vi "Report.vi"() -> ()   [LabVIEW 2017]
uses:
  <vilib>/Utility/miscctls.llb/LVRowAndColumnUnsignedTypeDef.ctl
  a160b8e7-0040-4e34-a052-5f80b3aab475.vi
  <vilib>/addons/database/Connection.llb/DB Tools Open Connec (String).vi
  <vilib>/Utility/file.llb/Write Delimited Spreadsheet (string).vi
  Global/Global 1.vi
  <vilib>/addons/database/NI_Database_API.lvlib
  <vilib>/Utility/NIReport.llb/NI_report.lvclass
  <vilib>/Utility/NIReport.llb/Append Text Table to Report (wrap).vi
panel:
  out "reposr save header":string[](array[string])
  in  "SELECT REPORT TYPE":string(combo)="WITH TRECIABILITY"
  out "error out":errorcluster
  in  "error in (no error)":errorcluster
  in  "GET REPORT":bool
  in  "EXIT":bool
  in  "EXPORT TO EXCEL":bool
  in  "TO":timestamp format="%<%x>T"
  in  "FROM":timestamp format="%<%x>T"
  in  "BARCODE":string
  in  "TYPE":string(combo)="DATE TIME"
  in  "STATION WISE":string(combo)="OP 10"
  out "Table":string[][](table)
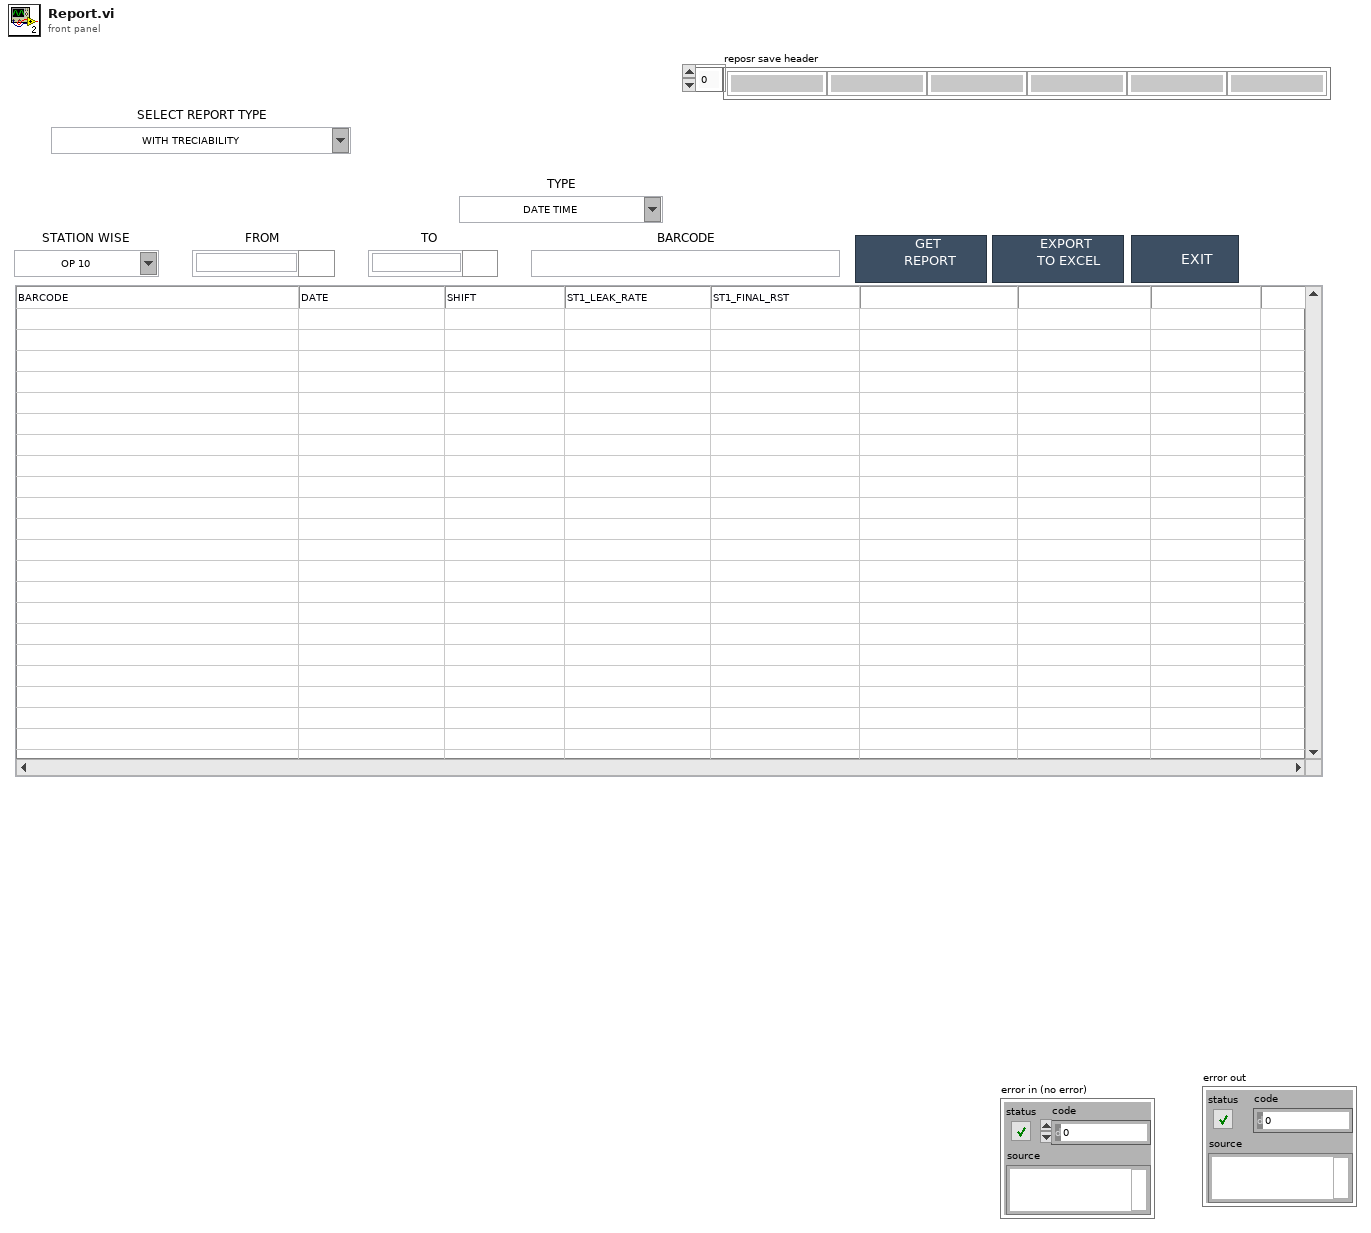
[diagram p1: front panel]
types:
  T1 = typedef "NI_Database_API.lvlib/Conn ObjectReference.ctl" = refnum<k1>
  T2 = typedef "LVRowAndColumnUnsignedTypeDef.ctl" = cluster{"Row":u32, "Column":u32}
  T3 = enum16{"Standard Report", "HTML", "Word", "Excel"}
  T4 = enum16{"maximized", "minimized", "normal", "no change"}
  T5 = typedef "LVRowAndColumnTypeDef.ctl" = cluster{"Row":i32, "Column":i32}
  T6 = enum32{"invalid app kind", "Development System", "Run Time System", "Student Edition", "Embedded LabVIEW", "Evaluation", "Custom"}
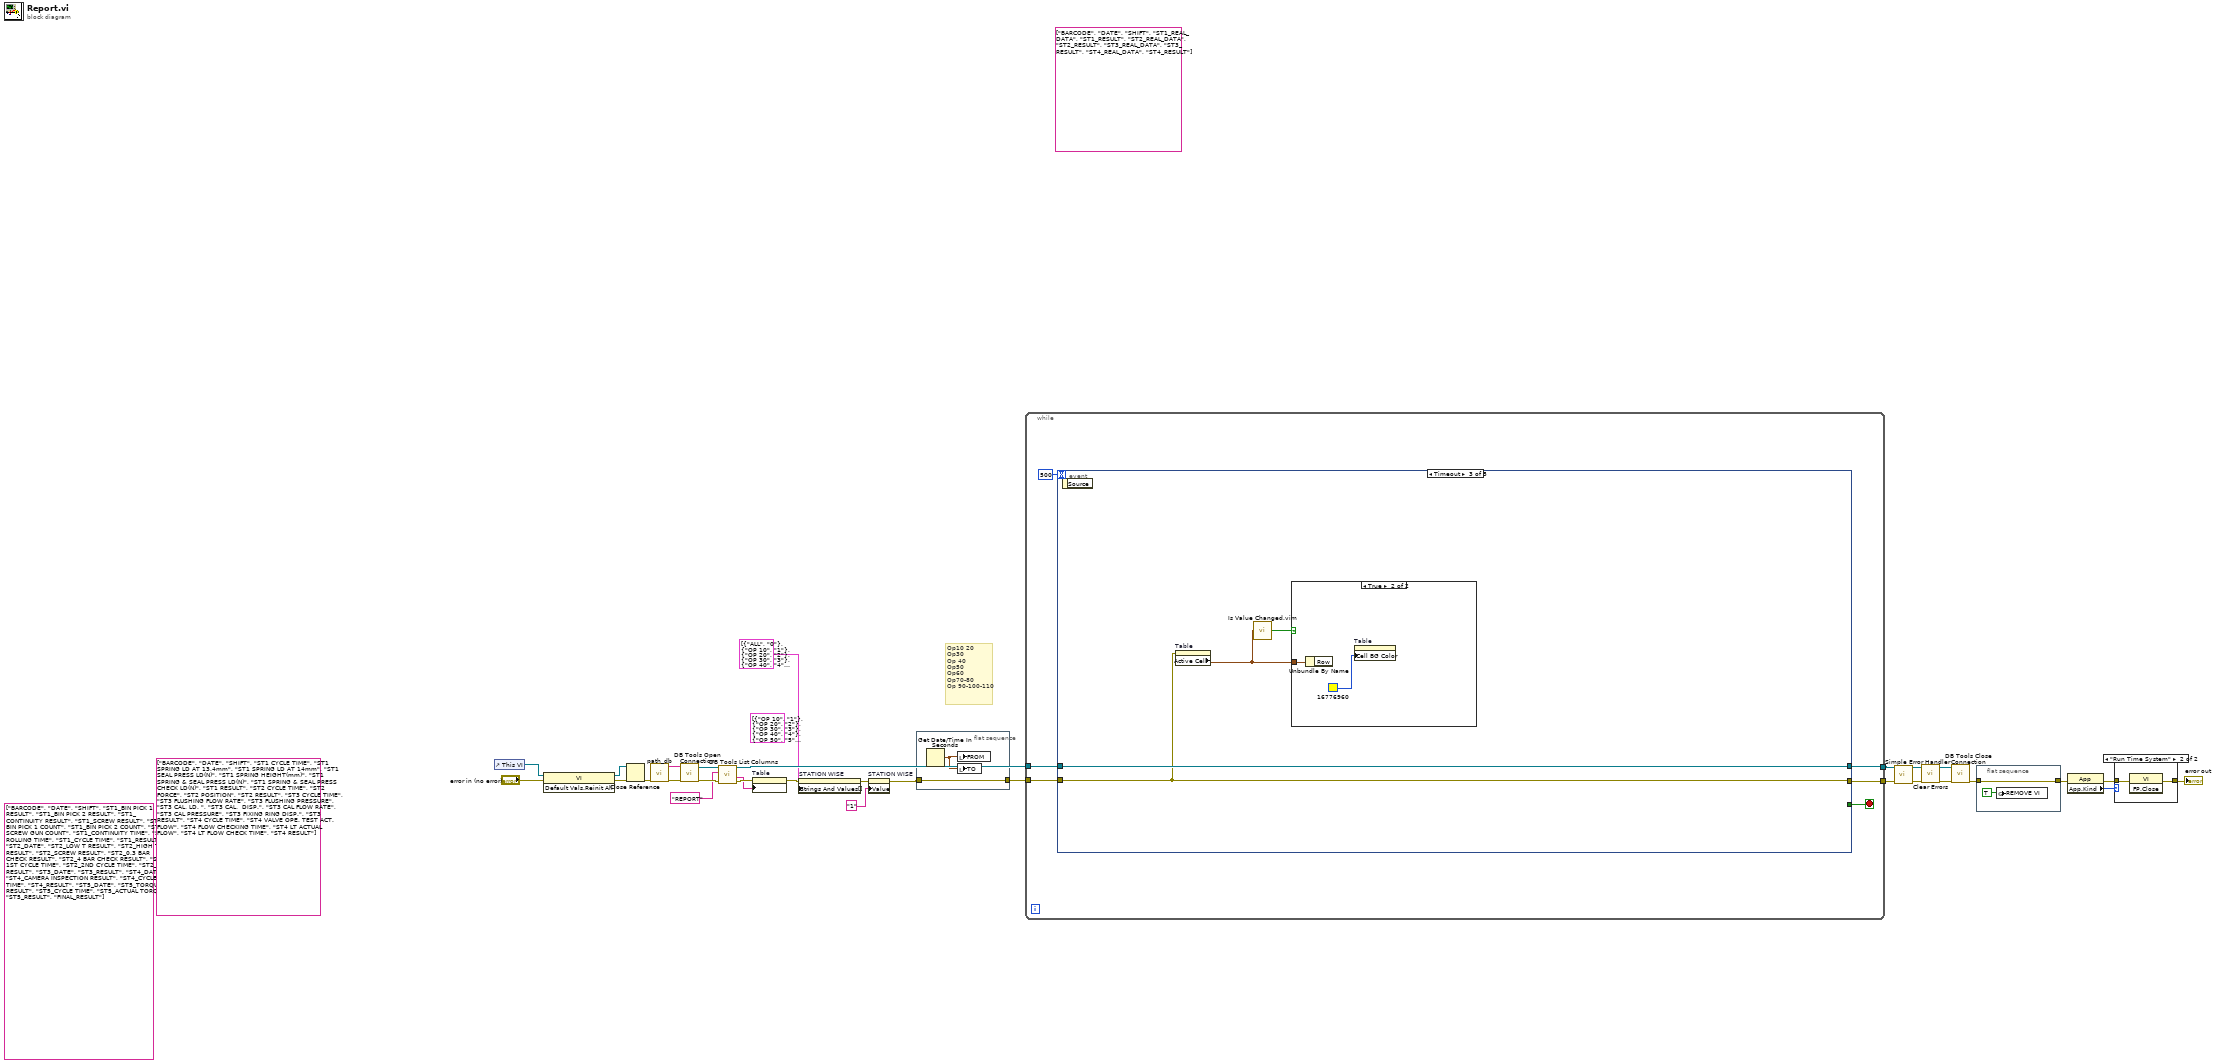
[diagram p0: block diagram]
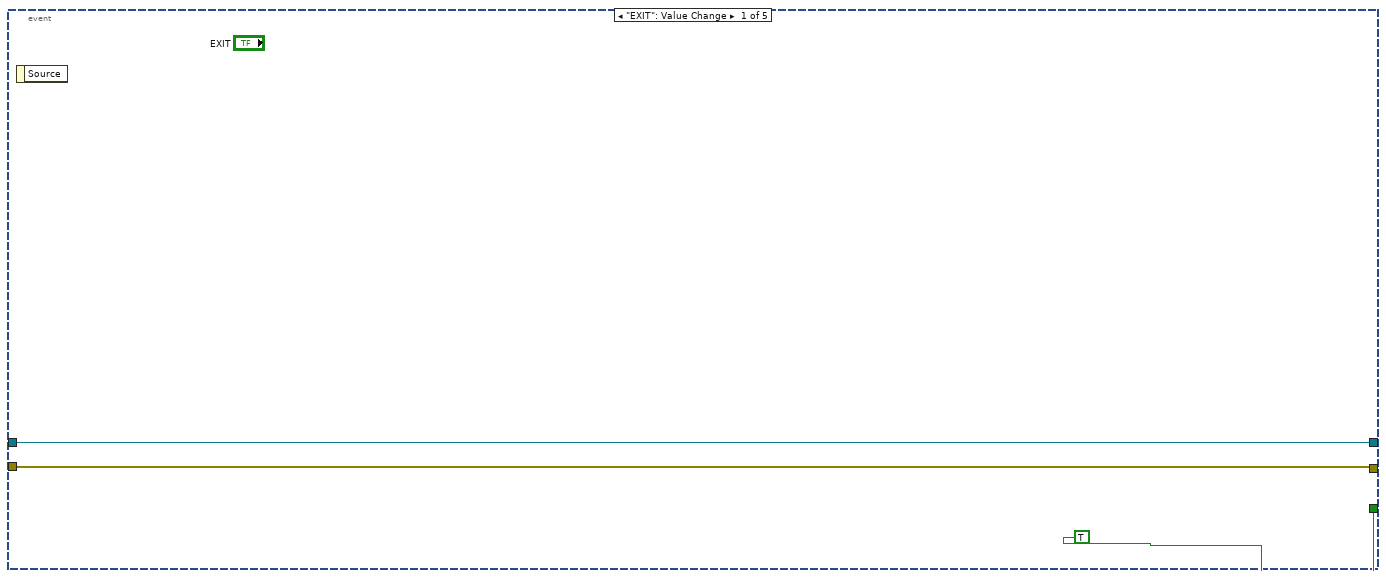
[diagram p2: hidden frame]
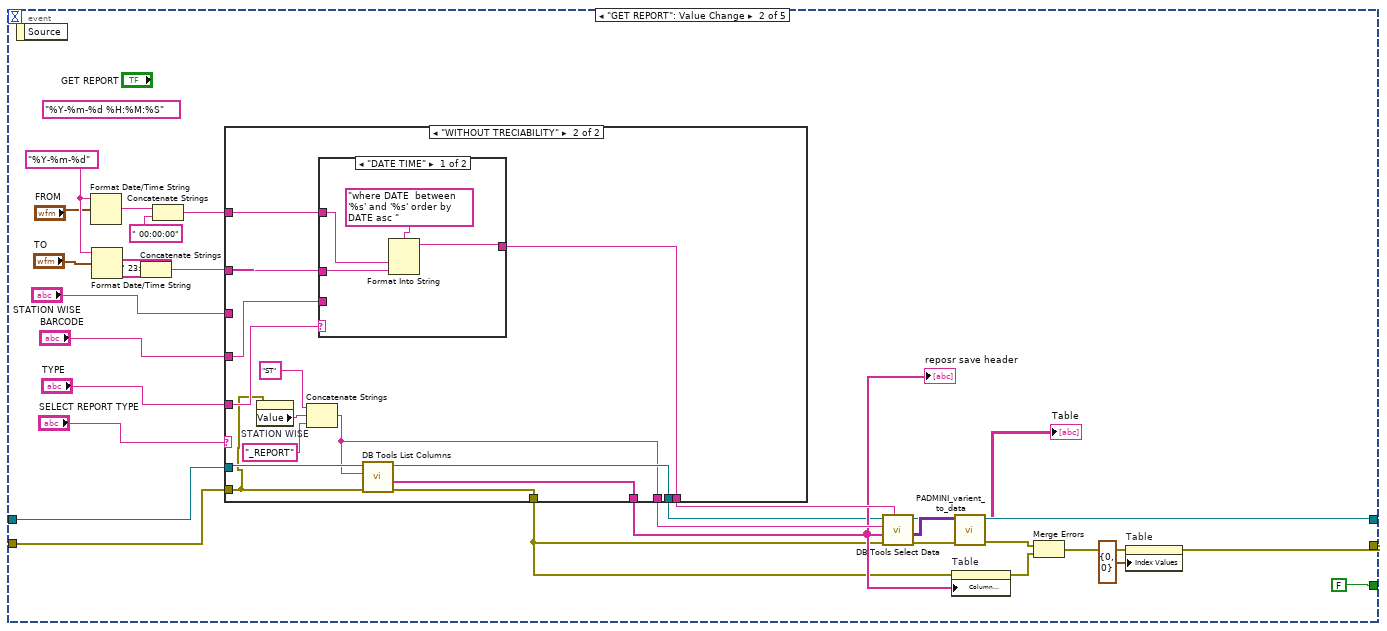
[diagram p3: hidden frame]
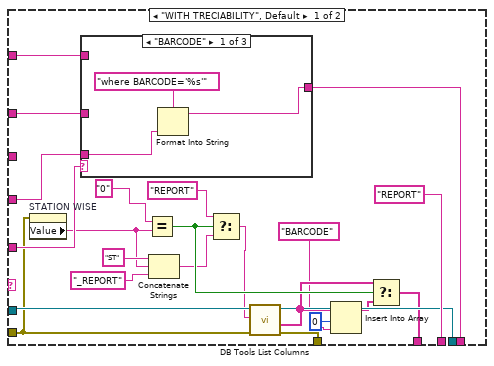
[diagram p4: hidden frame]
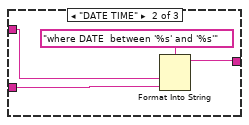
[diagram p5: hidden frame]
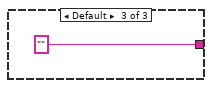
[diagram p6: hidden frame]
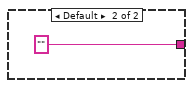
[diagram p7: hidden frame]
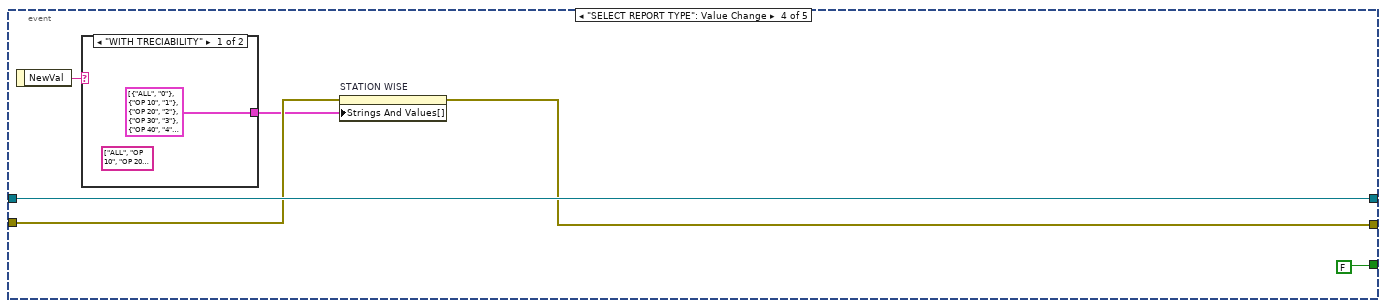
[diagram p9: hidden frame]
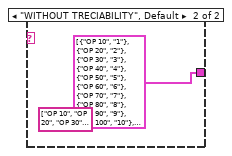
[diagram p10: hidden frame]
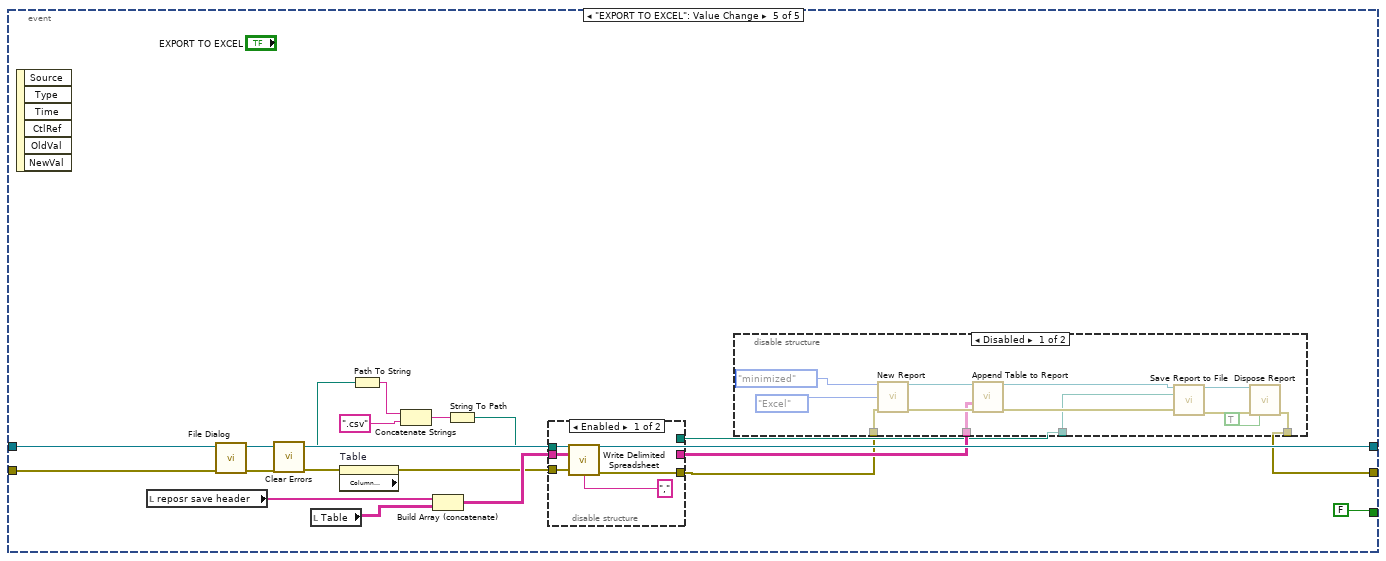
[diagram p11: hidden frame]
diagram:
  (unwired) cluster{"String":string, "Value":string}[] [{"String"="OP 10", "Value"="1"}, {"String"="OP 20", "Value"="2"}, {"String"="OP 30", "Value"="3"}, {"String"="OP 40", "Value"="4"}, {"String"="OP 50", "Value"="5"}, {"String"="OP 60", "Value"="6"}, {"String"="OP 70", "Value"="7"}, {"String"="OP 80", "Value"="8"}, {"String"="OP 90", "Value"="9"}, {"String"="OP 100", "Value"="10"}, {"String"="OP 110", "Value"="11"}] ("Strings And Values [] 2")
  (unwired) string[] ["BARCODE", "DATE", "SHIFT", "ST1_REAL_DATA", "ST1_RESULT", "ST2_REAL_DATA", "ST2_RESULT", "ST3_REAL_DATA", "ST3_RESULT", "ST4_REAL_DATA", "ST4_RESULT"]
  (unwired) string[] ["BARCODE", "DATE", "SHIFT", "ST1_BIN PICK 1 RESULT", "ST1_BIN PICK 2 RESULT", "ST1_CONTINUITY RESULT", "ST1_SCREW RESULT", "ST1_BIN PICK 1 COUNT", "ST1_BIN PICK 2 COUNT", "ST1_SCREW GUN COUNT", "ST1_CONTINUITY TIME", "ST1_ROLLING TIME", "ST1_CYCLE TIME", "ST1_RESULT", "ST2_DATE", "ST2_LOW T RESULT", "ST2_HIGH T RESULT", "ST2_SCREW RESULT", "ST2_0.3 BAR CHECK RESULT", "ST2_4 BAR CHECK RESULT", "ST2_1ST CYCLE TIME", "ST2_2ND CYCLE TIME", "ST2_RESULT", "ST3_DATE", "ST3_RESULT", "ST4_DATE", "ST4_CAMERA INSPECTION RESULT", "ST4_CYCLE TIME", "ST4_RESULT", "ST5_DATE", "ST5_TORQUE RESULT", "ST5_CYCLE TIME", "ST5_ACTUAL TORQUE", "ST5_RESULT", "FINAL_RESULT"]
  (unwired) string[] ["BARCODE", "DATE", "SHIFT", "ST1 CYCLE TIME", "ST1 SPRING LD AT 13.4mm", "ST1 SPRING LD AT 14mm", "ST1 SEAL PRESS LD(N)", "ST1 SPRING HEIGHT(mm)", "ST1 SPRING & SEAL PRESS LD(N)", "ST1 SPRING & SEAL PRESS CHECK LD(N)", "ST1 RESULT", "ST2 CYCLE TIME", "ST2 FORCE", "ST2 POSITION", "ST2 RESULT", "ST3 CYCLE TIME", "ST3 FLUSHING FLOW RATE", "ST3 FLUSHING PRESSURE", "ST3 CAL. LD. ", "ST3 CAL.  DISP.", "ST3 CAL FLOW RATE", "ST3 CAL PRESSURE", "ST3 FIXING RING DISP.", "ST3 RESULT", "ST4 CYCLE TIME", "ST4 VALVE OPE. TEST ACT. FLOW", "ST4 FLOW CHECKING TIME", "ST4 LT ACTUAL FLOW", "ST4 LT FLOW CHECK TIME", "ST4 RESULT"]
  # "Op10 20\nOp30\nOp 40\nOp50\nOp60\nOp70-80\nOp 90-100-110"
  n1 = control-ref of="This VI"() -> (w28:refnum<vi>)
  n2 = invoke class="VI" method="Default Vals.Reinit All"(reference=w28, error in="error in (no error)") -> (reference out=w26:refnum<vi>, error out=w25:errorcluster)  [unwired: 1 in, 1 out]
  n3 = Close Reference(reference=w26, error in (no error)=w25) -> (error out=w15:errorcluster)
  n4 = call "path_db.vi"("error in"=w15) -> ("error out"=w17:errorcluster, "resulting string"=w16:string)  [unwired: 9 in]
  n5 = call-poly <vilib>:"DB Tools Open Connection.vi"("error in (no error)"=w17, "connection information"=w16) -> ("error out"=w10:errorcluster, "connection reference"=w7:T1)  [unwired: 6 in]
  n6 = call <vilib>:"DB Tools List Columns.vi"("error in (no error)"=w10, "table"="REPORT", "connection reference"=w7) -> ("error out"=w9:errorcluster, "columns"=w6:string[], "connection reference out"=w8:T1)  [unwired: 1 in, 1 out]
  n7 = property on="Table" class="Tbl (strict)"(error in=w9, "Column Headers[]"=w6) -> (error out=w12:errorcluster)  [unwired: 1 in, 1 out]
  n8 = property on="STATION WISE" class="CmbBox"(error in=w12, "Strings And Values[]"=cluster{"String":string, "Value":string}[] [{"String"="ALL", "Value"="0"}, {"String"="OP 10", "Value"="1"}, {"String"="OP 20", "Value"="2"}, {"String"="OP 30", "Value"="3"}, {"String"="OP 40", "Value"="4"}, {"String"="OP 50", "Value"="5"}, {"String"="OP 60", "Value"="6"}, {"String"="OP 70", "Value"="7"}, {"String"="OP 80", "Value"="8"}, {"String"="OP 90", "Value"="9"}, {"String"="OP 100", "Value"="10"}, {"String"="OP 110", "Value"="11"}] ("Strings And Values [] 2")) -> (error out=w4:errorcluster)  [unwired: 1 in, 1 out]
  n9 = property on="STATION WISE" class="CmbBox"(error in=w4, "Value"="1") -> (error out=w3:errorcluster)  [unwired: 1 in, 1 out]
  n10 = flat-sequence {
    tunnel: w3 -> [w29]
    tunnel: [w29] -> w11
    frame #0 {
      n11 = Get Date/Time In Seconds() -> (seconds since 1Jan1904=w30:timestamp)
      n12 = local write "FROM"(w30) -> ()
      n13 = local write "TO"(w30) -> ()
    }
  }
  n14 = while {
    tunnel: [w33] -> w18
    tunnel: w11 -> [w35]
    tunnel: w8 -> [w34]
    tunnel: [w32] -> w13
    stop <- w36 stop-if-true
    n15 = event shown="[2] Timeout" {
      selector: _ -> [_ _ _ _ _]
      dyn-events: _ -> [_ _ _ _ _]
      timeout: 500 -> [_ _ _ _ _]
      tunnel: [TRUE FALSE _ FALSE FALSE] -> w36
      tunnel: w35 -> [w37 w46 w120 w129 w139]
      tunnel: w34 -> [w38 w44 w123 w131 w150]
      tunnel: [w38 w52 w123 w131 w150] -> w32
      tunnel: [w37 w53 w120 w126 w136] -> w33
      event "EXIT": Value Change {
        n16 = event-data() -> ()  [unwired: 1 in, 1 out]
      }
      event "GET REPORT": Value Change {
        (unwired) "%Y-%m-%d %H:%M:%S" ("time format string (%c)")
        w66 = "%Y-%m-%d" ("time format string (%c)")
        n17 = event-data() -> ()  [unwired: 1 in, 1 out]
        n18 = Format Date/Time String(time format string (%c)=w66, seconds (now)="FROM") -> (date/time string=w60:string)  [unwired: 1 in]
        n19 = Format Date/Time String(time format string (%c)=w66, seconds (now)="TO") -> (date/time string=w57:string)  [unwired: 1 in]
        n20 = Concatenate Strings(w57, " 23:59:59" ("time format string (%c)")) -> (w56:string)
        n21 = Concatenate Strings(w60, " 00:00:00" ("time format string (%c)")) -> (w59:string)
        n22 = case shown="\"WITHOUT TRECIABILITY\"" "SELECT REPORT TYPE" {
          tunnel: "TYPE" -> [w92 w114]
          tunnel: [w91 w113] -> w68
          tunnel: "BARCODE" -> [w90 w112]
          tunnel: w59 -> [w89 w111]
          tunnel: w56 -> [w88 w107]
          tunnel: "STATION WISE" -> [_ _]
          tunnel: ["REPORT" w102] -> w47
          tunnel: w46 -> [w70 w101]
          tunnel: [w84 w106] -> w40
          tunnel: [w80 w105] -> w45
          tunnel: w44 -> [w86 w104]
          tunnel: [w85 w103] -> w43
          frame "WITH TRECIABILITY", Default {
            n23 = property on="STATION WISE" class="CmbBox"(error in=w70) -> ("Value"=w71:string)  [unwired: 1 in, 2 out]
            n24 = case shown="\"BARCODE\"" w92 {
              tunnel: [w94 w98 ""] -> w91
              tunnel: w90 -> [w93 _ _]
              tunnel: w89 -> [_ w97 _]
              tunnel: w88 -> [_ w96 _]
              frame "BARCODE" {
                n25 = Format Into String(format string="where BARCODE='%s'", w93) -> (resulting string=w94:string)  [unwired: 2 in, 1 out]
              }
              frame "DATE TIME" {
                n26 = Format Into String(format string="where DATE  between '%s' and '%s'", w97, w96) -> (resulting string=w98:string)  [unwired: 2 in, 1 out]
              }
              frame Default {
              }
            }
            n27 = Equal?(x="0", y=w71) -> (x = y?=w82:bool)
            n28 = Concatenate Strings("ST", w71, "_REPORT") -> (w74:string)
            n29 = Select(t="REPORT", s=w82, f=w74) -> (s? t:f=w81:string)
            n30 = call <vilib>:"DB Tools List Columns.vi"("error in (no error)"=w70, "table"=w81, "connection reference"=w86) -> ("error out"=w84:errorcluster, "columns"=w79:string[], "connection reference out"=w85:T1)  [unwired: 1 in, 1 out]
            n31 = Insert Into Array(array=w79, index=0, new element="BARCODE" ("String")) -> (w77:string[])
            n32 = Select(t=w79, s=w82, f=w77) -> (s? t:f=w80:string[])
          }
          frame "WITHOUT TRECIABILITY" {
            n33 = property on="STATION WISE" class="CmbBox"(error in=w101) -> ("Value"=w110:string)  [unwired: 1 in, 2 out]
            n34 = Concatenate Strings("ST", w110, "_REPORT") -> (w102:string)
            n35 = case shown="\"DATE TIME\"" w114 {
              tunnel: [w118 ""] -> w113
              tunnel: w112 -> [_ _]
              tunnel: w111 -> [w117 _]
              tunnel: w107 -> [w116 _]
              frame "DATE TIME" {
                n36 = Format Into String(format string="where DATE  between '%s' and '%s' order by DATE asc ", w117, w116) -> (resulting string=w118:string)  [unwired: 2 in, 1 out]
              }
              frame Default {
              }
            }
            n37 = call <vilib>:"DB Tools List Columns.vi"("error in (no error)"=w101, "table"=w102, "connection reference"=w104) -> ("error out"=w106:errorcluster, "columns"=w105:string[], "connection reference out"=w103:T1)  [unwired: 1 in, 1 out]
          }
        }
        "reposr save header" <- w45
        n38 = call <vilib>:"DB Tools Select Data.vi"("condition"=w68, "error in (no error)"=w40, "columns"=w45, "table"=w47, "connection reference"=w43) -> ("error out"=w50:errorcluster, "data"=w55:variant[][], "connection reference out"=w52:T1)  [unwired: 1 in]
        n39 = property on="Table" class="Tbl (strict)"(error in=w40, "Column Headers[]"=w45) -> (error out=w49:errorcluster)  [unwired: 1 in, 1 out]
        n40 = call "PADMINI_varient_to_data.vi"("error in (no error)"=w50, "data"=w55) -> ("error out"=w48:errorcluster, "Array"=→"Table":string[][])  [unwired: 8 in]
        n41 = Merge Errors(w48, w49) -> (w54:errorcluster)
        n42 = property on="Table" class="Tbl (strict)"(error in=w54, "Index Values"=T2 {"Row"=0, "Column"=0}) -> (error out=w53:errorcluster)  [unwired: 1 in, 1 out]
      }
      event Timeout {
        n43 = event-data() -> ()  [unwired: 1 in, 1 out]
        n44 = property on="Table" class="Tbl (strict)"(error in=w120) -> ("Active Cell"=w122:T5)  [unwired: 1 in, 2 out]
        n45 = call "Is Value Changed.vim"("value"=w122) -> ("changed or first call?"=w121:bool)
        n46 = case shown="True" w121 {
          tunnel: w122 -> [_ w125]
          frame False {
          }
          frame True {
            n47 = Unbundle By Name(w125) -> ()  [unwired: 1 out]
            n48 = property on="Table" class="Tbl (strict)"("Cell BG Color"=u32 16776960) -> ()  [unwired: 2 in, 2 out]
          }
        }
      }
      event "SELECT REPORT TYPE": Value Change {
        n49 = event-data() -> ("NewVal"=w130:string)  [unwired: 1 in]
        n50 = case shown="\"WITH TRECIABILITY\"" w130 {
          tunnel: [cluster{"String":string, "Value":string}[] [{"String"="ALL", "Value"="0"}, {"String"="OP 10", "Value"="1"}, {"String"="OP 20", "Value"="2"}, {"String"="OP 30", "Value"="3"}, {"String"="OP 40", "Value"="4"}, {"String"="OP 50", "Value"="5"}, {"String"="OP 60", "Value"="6"}, {"String"="OP 70", "Value"="7"}, {"String"="OP 80", "Value"="8"}, {"String"="OP 90", "Value"="9"}, {"String"="OP 100", "Value"="10"}, {"String"="OP 110", "Value"="11"}] ("Strings And Values [] 2") cluster{"String":string, "Value":string}[] [{"String"="OP 10", "Value"="1"}, {"String"="OP 20", "Value"="2"}, {"String"="OP 30", "Value"="3"}, {"String"="OP 40", "Value"="4"}, {"String"="OP 50", "Value"="5"}, {"String"="OP 60", "Value"="6"}, {"String"="OP 70", "Value"="7"}, {"String"="OP 80", "Value"="8"}, {"String"="OP 90", "Value"="9"}, {"String"="OP 100", "Value"="10"}, {"String"="OP 110", "Value"="11"}] ("Strings And Values [] 2")] -> w127
          frame "WITH TRECIABILITY" {
            (unwired) string[] ["ALL", "OP 10", "OP 20", "OP 30", "OP 40", "OP 50", "OP 60", "OP 70", "OP 80", "OP 90", "OP 100", "OP 110"] ("Strings []")
          }
          frame "WITHOUT TRECIABILITY", Default {
            (unwired) string[] ["OP 10", "OP 20", "OP 30", "OP 40", "OP 50", "OP 60", "OP 70", "OP 80", "OP 90", "OP 100", "OP 110"] ("Strings []")
          }
        }
        n51 = property on="STATION WISE" class="CmbBox"(error in=w129, "Strings And Values[]"=w127) -> (error out=w126:errorcluster)  [unwired: 1 in, 1 out]
      }
      event "EXPORT TO EXCEL": Value Change {
        n52 = event-data() -> ()  [unwired: 1 in, 6 out]
        n53 = local read "reposr save header"() -> (w134:string[])
        n54 = call "File Dialog"("error in"=w139) -> ("selected path"=w148:path, "error out"=w149:errorcluster)  [unwired: 11 in, 2 out]
        n55 = call <vilib>:"Clear Errors.vi"("error in (no error)"=w149) -> ("error out"=w142:errorcluster)  [unwired: 5 in, 1 out]
        n56 = local read "Table"() -> (w151:string[][])
        n57 = property on="Table" class="Tbl (strict)" props=["Column Headers[]"](error in=w142) -> (error out=w141:errorcluster)  [unwired: 1 in, 2 out]
        n58 = Path To String(path=w148) -> (string=w147:string)
        n59 = Concatenate Strings(w147, ".csv" ("string")) -> (w145:string)
        n60 = Build Array (concatenate)(w134, w151) -> (w143:string[][])
        n61 = String To Path(string=w145) -> (path=w144:path)
        n62 = disable-structure shown="Enabled" {
          disable-tunnel: w144 -> [w170 w171]
          disable-tunnel: [w169 w173] -> w135
          disable-tunnel: w143 -> [w168 w172]
          disable-tunnel: w141 -> [w166 w173]
          disable-tunnel: [_ w172] -> w138
          disable-tunnel: [_ w171] -> w137
          frame Enabled {
            n63 = call-poly <vilib>:"Write Delimited Spreadsheet.vi"("file path (dialog if empty)"=w170, "2D data"=w168, "error in (no error)"=w166, "delimiter (\\t)"="," ("delimiter (\\t)")) -> ("error out"=w169:errorcluster)  [unwired: 10 in, 1 out]
          }
          frame Disabled {
          }
        }
        n64 = disable-structure shown="Disabled" {
          disable-tunnel: w138 -> [w155 _]
          disable-tunnel: w137 -> [w154 _]
          disable-tunnel: [w153 w165] -> w136
          disable-tunnel: w135 -> [w152 w165]
          frame Disabled {
            n65 = call <vilib>:"New Report.vi"("window state (normal)"=T4."minimized", "report type"=T3."Excel", "error in (no error)"=w152) -> ("report out"=w162:refnum<class "NI_report.lvclass">, "error out"=w161:errorcluster)  [unwired: 11 in]
            n66 = call-poly <vilib>:"Append Table to Report.vi"("report in"=w162, "text data"=w155, "error in (no error)"=w161) -> ("report out"=w158:refnum<class "NI_report.lvclass">, "error out"=w160:errorcluster)  [unwired: 9 in, 2 out]
            n67 = call-dynamic "Save Report to File.vi"("report in"=w158, "report file path"=w154, "error in (no error)"=w160) -> ("report out"=w157:refnum<class "NI_report.lvclass">, "error out"=w159:errorcluster)  [unwired: 11 in]
            n68 = call-dynamic "Dispose Report.vi"("report in"=w157, "error in (no error)"=w159, "close report? (T)"=TRUE) -> ("error out"=w153:errorcluster)  [unwired: 12 in]
          }
          frame Enabled {
          }
        }
      }
    }
  }
  n69 = call <vilib>:"Simple Error Handler.vi"("error in (no error)"=w18) -> ("error out"=w24:errorcluster)  [unwired: 4 in, 4 out]
  n70 = call <vilib>:"Clear Errors.vi"("error in (no error)"=w24) -> ("error out"=w23:errorcluster)  [unwired: 5 in, 1 out]
  n71 = call <vilib>:"DB Tools Close Connection.vi"("error in (no error)"=w23, "connection reference"=w13) -> ("error out"=w14:errorcluster)  [unwired: 5 in]
  n72 = flat-sequence {
    tunnel: [w175] -> w22
    tunnel: w14 -> [w175]
    frame #0 {
      n73 = global write "Global 1.vi" "REMOVE VI"(TRUE ("REMOVE VI")) -> ()
    }
  }
  n74 = property class="App"(error in=w22) -> (error out=w21:errorcluster, "App.Kind"=w20:T6)  [unwired: 1 in, 1 out]
  n75 = case shown="\"Run Time System\"" w20 {
    tunnel: w21 -> [w176 w178]
    tunnel: [w176 w177] -> w19
    frame "Development System", Default {
    }
    frame "Run Time System" {
      n76 = invoke class="VI" method="FP.Close"(error in=w178) -> (error out=w177:errorcluster)  [unwired: 2 in, 2 out]
    }
  }
  "error out" <- w19
